vi "testAttributeQuotesSingleWithDoubleInside.vi"(8 "error in (no error)":errorcluster, 11 "TestCase in":refnum<class "EasyXMLTest.lvclass">) -> (0 "error out":errorcluster, 3 "TestCase out":refnum<class "EasyXMLTest.lvclass">)   [LabVIEW 2013, in "EasyXMLTest.lvclass"]
doc: "Verify that error in is not overwritten"
uses:
  EasyXMLTest.lvclass
panel:
  out "Produced Data":variant
  out "Input Data":variant
  out "XML String":string
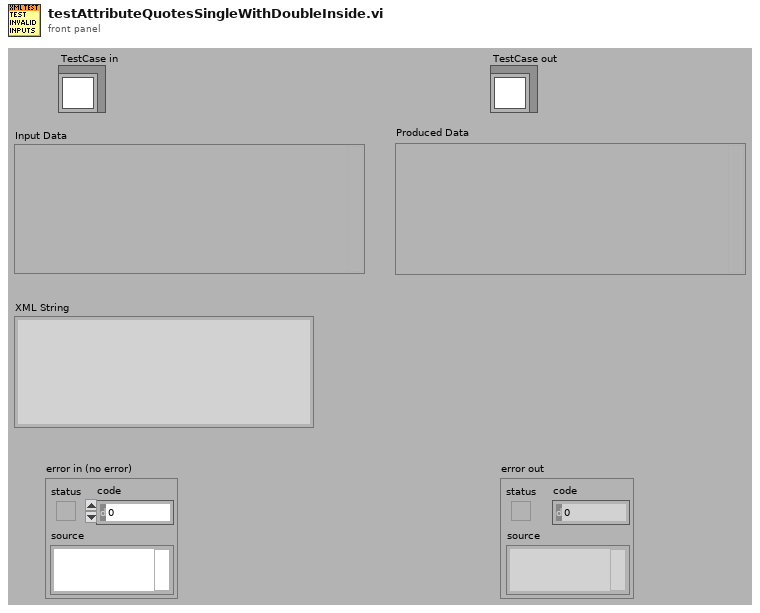
[diagram p1: front panel]
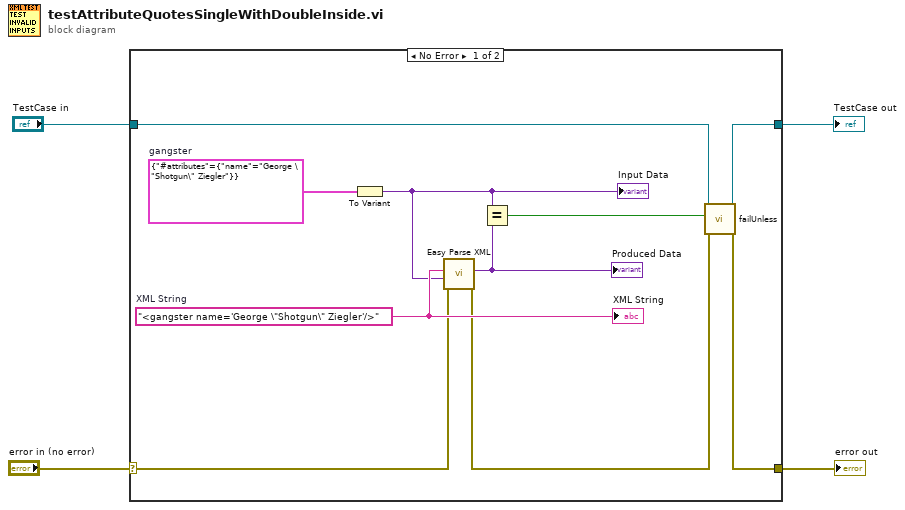
[diagram p0: block diagram]
diagram:
  n1 = case shown="No Error" "error in (no error)" {
    selector: "error in (no error)" -> [w7 w16]
    tunnel: [w10 w16] -> w2
    tunnel: [w8 w15] -> w1
    tunnel: "TestCase in" -> [w9 w15]
    frame No Error {
      w5 = cluster{"#attributes":cluster{"name":string}} {"#attributes"={"name"="George \"Shotgun\" Ziegler"}}  # gangster
      w14 = "<gangster name='George \"Shotgun\" Ziegler'/>"  # XML String
      n2 = To Variant(anything=w5) -> (Variant=w13:variant)
      "Input Data" <- w13
      n3 = call "Easy Parse XML.vi"("error in (no error)"=w7, "LabVIEW Data (Type)"=w13, "XML String"=w14) -> ("error out"=w6:errorcluster, "LabVIEW Data"=w12:variant)  [unwired: 7 in]
      "Produced Data" <- w12
      n4 = Equal?(x=w13, y=w12) -> (x = y?=w11:bool)
      n5 = call-dynamic "failUnless.vi"("error in (no error)"=w6, "pass"=w11, "TestCase in"=w9) -> ("error out"=w10:errorcluster, "TestCase out"=w8:refnum<class "EasyXMLTest.lvclass">)  [unwired: 7 in]
      "XML String" <- w14
    }
    frame Error {
    }
  }
  "error out" <- w2
  "TestCase out" <- w1
